vi "1_3.vi"() -> ()   [LabVIEW 2010]
panel:
  in  "OK Button":bool
  out "Numeric":i32
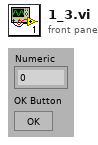
[diagram p1: front panel]
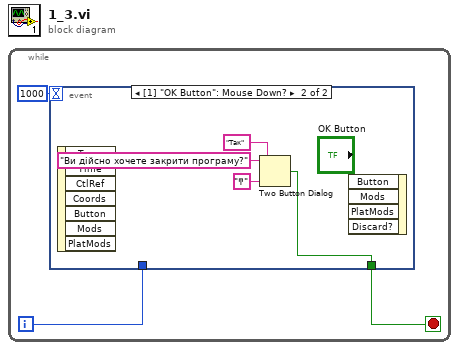
[diagram p0: block diagram]
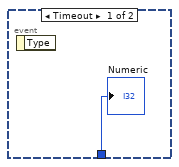
[diagram p2: hidden frame]
diagram:
  n1 = while {
    i -> [w1]
    stop <- w2 stop-if-true
    n2 = event shown="[1] \"OK Button\": Mouse Down?" {
      selector: _ -> [_ _]
      dyn-events: _ -> [_ _]
      timeout: 1000 -> [_ _]
      tunnel: [_ w5] -> w2
      tunnel: w1 -> [w4 _]
      event Timeout {
        n3 = event-data() -> ()  [unwired: 1 in, 1 out]
        "Numeric" <- w4
      }
      event "OK Button": Mouse Down? {
        n4 = event-data() -> ()  [unwired: 1 in, 7 out]
        n5 = Two Button Dialog(message="Ви дійсно хочете закрити програму?", 1:"ͳ" ("F button name (\"Cancel\")"), 2:"Так" ("T button name (\"OK\")")) -> (T button?=w5:bool)
        n6 = event-data() -> ()  [unwired: 5 in, 1 out]
      }
    }
  }
